vi "Get TDMS File Directory.vi"(0 "tdms file directory in":path, 5 "calling vi path":path) -> (4 "tdms file directory out":path)   [LabVIEW 2023, in "GettingStarted_Common_148X_Host.lvlib"]
uses:
  GettingStarted_Common_148X_Host.lvlib
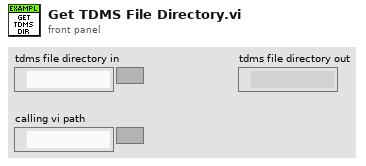
[diagram p1: front panel]
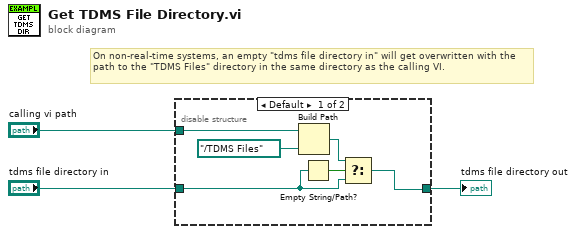
[diagram p0: block diagram]
diagram:
  # "On non-real-time systems, an empty \"tdms file directory in\" will get overwritten with the path to the \"TDMS Files\" directory in the same directory as the calling VI."
  n1 = disable-structure shown="Default" {
    disable-tunnel: [w9 w10] -> w2
    disable-tunnel: "tdms file directory in" -> [w6 w10]
    disable-tunnel: "calling vi path" -> [w5 _]
    frame condition #0 (active) {
      n2 = Build Path(base path=w5, name or relative path=path "../TDMS Files") -> (appended path=w8:path)
      n3 = Empty String/Path?(string/path=w6) -> (empty?=w7:bool)
      n4 = Select(t=w8, s=w7, f=w6) -> (s? t:f=w9:path)
    }
    frame condition #1 {
    }
  }
  "tdms file directory out" <- w2
